vi "Multicast4.vi"(8 "error in":errorcluster, 9 "VersionControl":bool, 11 "type_version":u32 format="%08x") -> (0 "error out":errorcluster, 1 "selDevice":T1, 2 "tblT":string[][](table) caption="Найденные устройства. (Выберите устройство к которому следует подключиться).", 3 "Cancel":bool, 4 "selIPhex":u32 format="%x", 5 "foundDevices":T1[](array[typedef]))   [LabVIEW 2017, in "LV_Unicorn.lvlib"]
uses:
  LV_Unicorn.lvlib
  Control/AnswerUDP.ctl
  <vilib>/Utility/miscctls.llb/LVRowAndColumnTypeDef.ctl
  Common/GlobalMulticast.vi
panel:
  in  "Listbox":i32(listbox)
  in  "Sel":bool
  in  "Cancel":bool
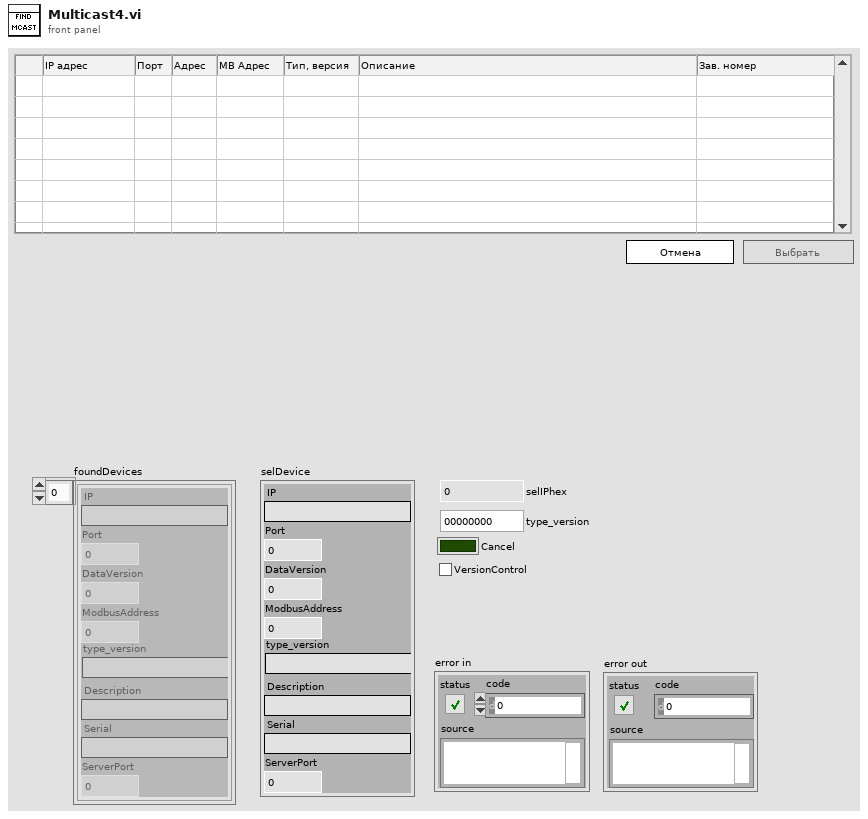
[diagram p1: front panel]
types:
  T1 = typedef "LV_Unicorn.lvlib/AnswerUDP.ctl" = cluster{"IP":string, "Port":u16, "DataVersion":u16, "ModbusAddress":i32, "type_version":string, "Description":string, "Serial":string, "ServerPort":u16}
  T2 = typedef "LVRowAndColumnTypeDef.ctl" = cluster{"Row":i32, "Column":i32}
  T3 = enum8{"Enabled", "Disabled", "Disabled and Grayed Out"}
  T4 = enum32{"Invalid", "Standard", "Closed", "Hidden", "Minimized", "Maximized"}
  T5 = enum32{"Bad", "Idle", "Run top level", "Running"}
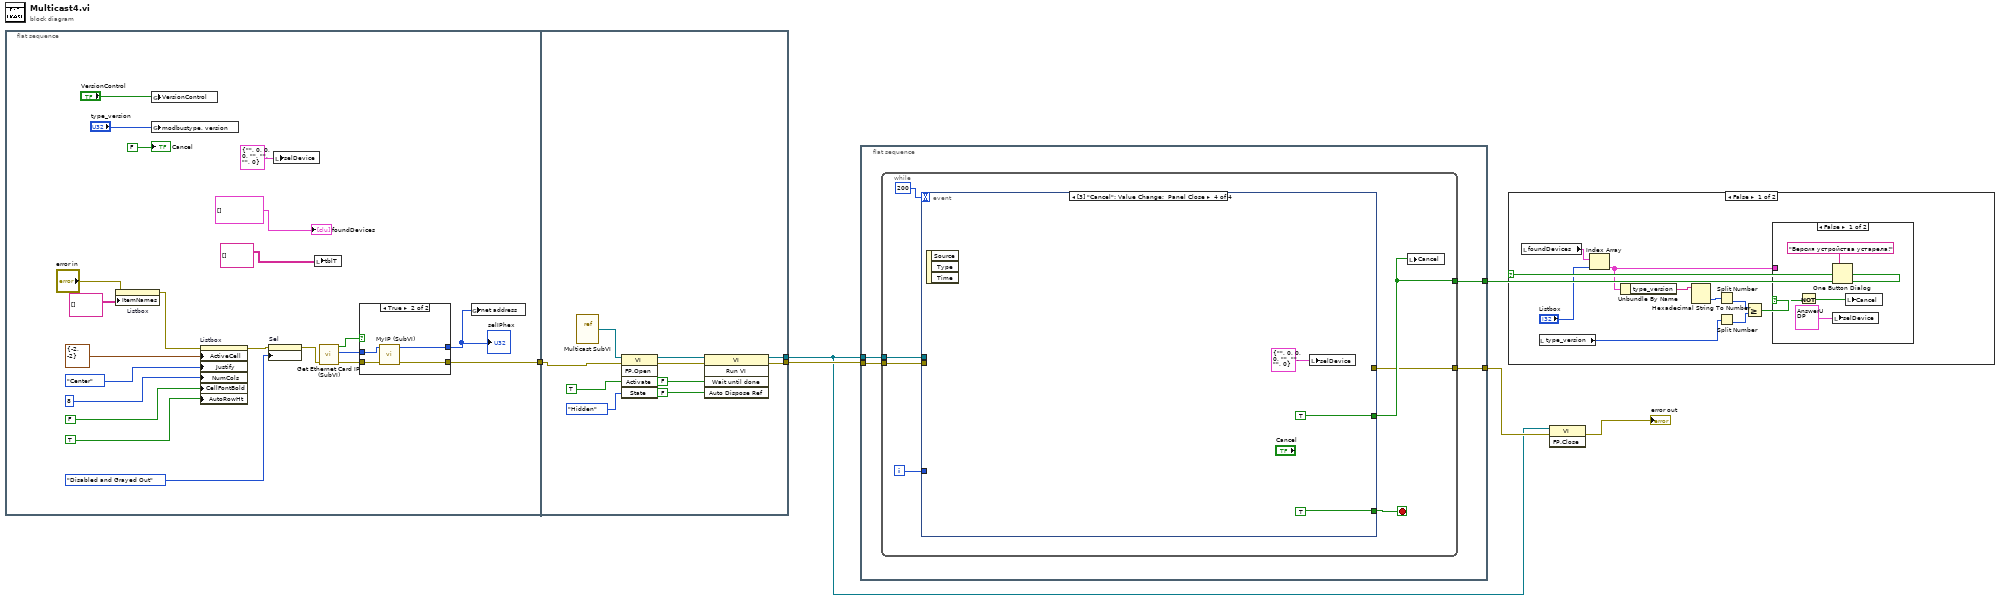
[diagram p0: block diagram]
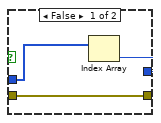
[diagram p2: hidden frame]
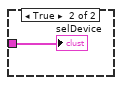
[diagram p3: hidden frame]
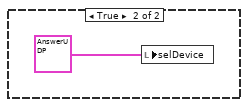
[diagram p4: hidden frame]
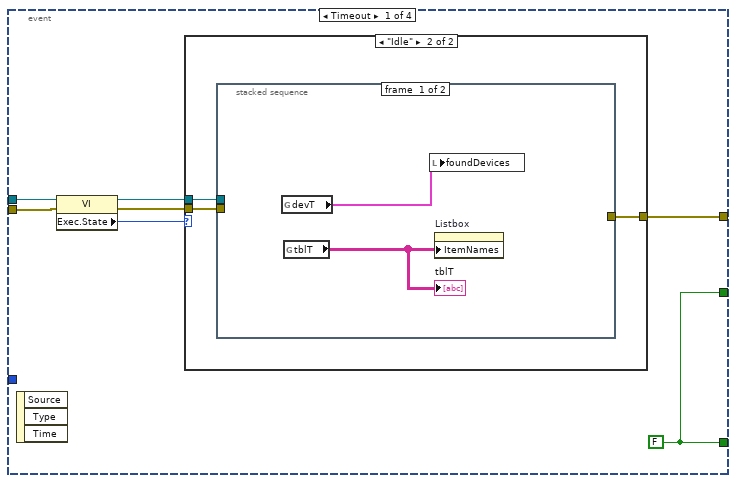
[diagram p5: hidden frame]
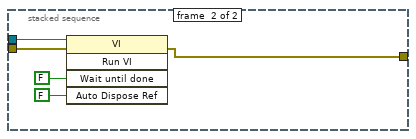
[diagram p7: hidden frame]
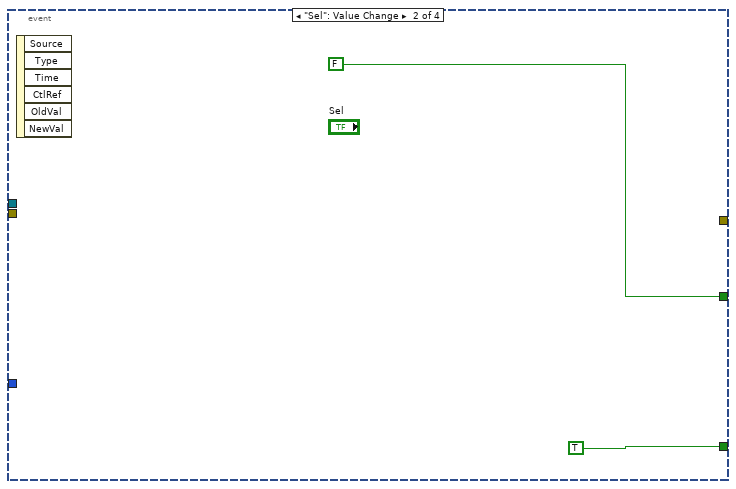
[diagram p8: hidden frame]
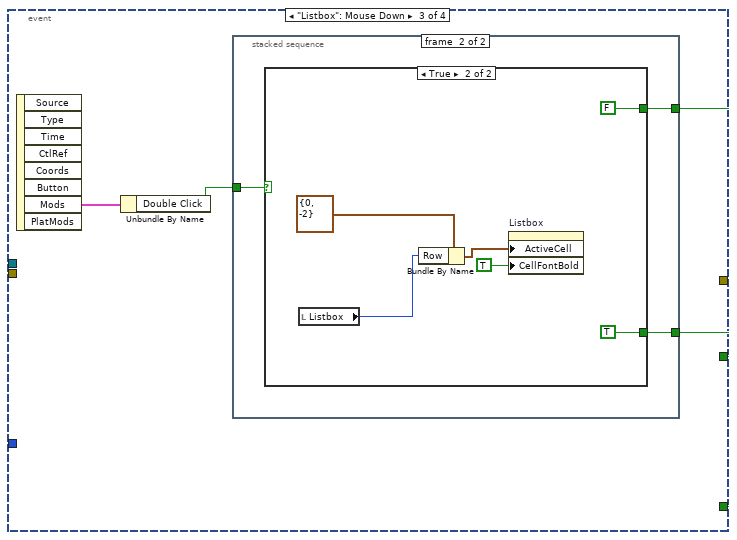
[diagram p9: hidden frame]
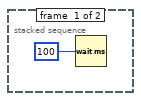
[diagram p10: hidden frame]
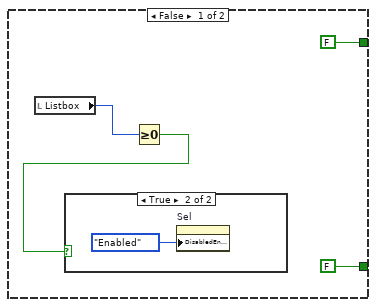
[diagram p11: hidden frame]
diagram:
  n1 = flat-sequence {
    tunnel: [w24] -> w4
    tunnel: [w44] -> w1
    tunnel: [w43] -> w5
    tunnel: w4 -> [w38]
    frame #0 {
      n2 = property on="Listbox" class="MCListbox (strict)"(error in="error in", "ItemNames"=string[][] [] ("Item Names")) -> (error out=w9:errorcluster)  [unwired: 1 in, 1 out]
      n3 = global write "GlobalMulticast.vi" "VersionControl"("VersionControl") -> ()
      n4 = global write "GlobalMulticast.vi" "modbustype, version"("type_version") -> ()
      n5 = property on="Listbox" class="MCListbox (strict)"(error in=w9, "ActiveCell"=T2 {"Row"=-2, "Column"=-2} ("Active Cell:Active Cell"), "Justify"=enum16{"Left", "Center", "Right"}."Center" ("Active Cell:Cell Justification"), "NumCols"=u32 8 ("Number of Columns"), "CellFontBold"=FALSE ("Active Cell:Cell Font:Bold"), "AutoRowHt"=TRUE ("Autosizing Row Height")) -> (error out=w10:errorcluster)  [unwired: 1 in, 1 out]
      n6 = property on="Sel" class="Bool"(error in=w10, "DisabledEnum"=T3."Disabled and Grayed Out" ("Disabled")) -> (error out=w16:errorcluster)  [unwired: 1 in, 1 out]
      n7 = local write "selDevice"(T1 {"IP"="", "Port"=0, "DataVersion"=0, "ModbusAddress"=0, "type_version"="", "Description"="", "Serial"="", "ServerPort"=0} ("selDevicesT")) -> ()
      n8 = local write "tblT"(string[][] [] ("table")) -> ()
      n9 = call "Get Ethernet Card IP (SubVI).vi"("error in (no error)"=w16) -> ("error out"=w28:errorcluster, "IP_hex"=w27:u32[], "FinIPMore1"=w26:bool)  [unwired: 8 in]
      n10 = case shown="True" w26 {
        tunnel: [w30 w33] -> w25
        tunnel: w28 -> [w29 w35]
        tunnel: w27 -> [w31 w34]
        tunnel: [w29 w32] -> w24
        frame False {
          n11 = Index Array(array=w31) -> (element=w30:u32)  [unwired: 1 in]
        }
        frame True {
          n12 = call "MyIP (SubVI).vi"("error in (no error)"=w35, "IPArray"=w34) -> ("error out"=w32:errorcluster, "Sel_IP_hex"=w33:u32)  [unwired: 8 in]
        }
      }
      "selIPhex" <- w25
      n13 = global write "GlobalMulticast.vi" "net address"(w25) -> ()
      "foundDevices" <- T1[] [] ("devices")
      "Cancel" <- FALSE ("Stop")
    }
    frame #1 {
      n14 = vi-ref "Multicast SubVI.vi"() -> (w41:refnum<vi>)
      n15 = invoke class="VI" method="FP.Open"(reference=w41, error in=w38, "Activate"=TRUE ("Activate?"), "State"=T4."Hidden") -> (reference out=w40:refnum<vi>, error out=w39:errorcluster)  [unwired: 1 in, 3 out]
      n16 = invoke class="VI" method="Run VI"(reference=w40, error in=w39, "Wait until done"=FALSE ("Wait Until Done"), "Auto Dispose Ref"=FALSE ("Auto Dispose Reference")) -> (reference out=w44:refnum<vi>, error out=w43:errorcluster)  [unwired: 1 in, 3 out]
    }
  }
  n17 = flat-sequence {
    tunnel: [w49] -> w6
    tunnel: w1 -> [w48]
    tunnel: w5 -> [w47]
    tunnel: [w46] -> w3
    frame #0 {
      n18 = while {
        tunnel: [w54] -> w49
        tunnel: w48 -> [w53]
        tunnel: w47 -> [w52]
        tunnel: [w50] -> w46
        i -> [w55]
        stop <- w56 stop-if-true
        n19 = event shown="[3] \"Cancel\": Value Change;  Panel Close" {
          selector: _ -> [_ _ _ _]
          dyn-events: _ -> [_ _ _ _]
          timeout: 200 -> [_ _ _ _]
          tunnel: [w63 TRUE w79 TRUE] -> w56
          tunnel: w55 -> [_ _ _ _]
          tunnel: [w63 FALSE ("Cancel") w78 TRUE ("Cancel")] -> w54
          tunnel: w53 -> [w62 _ _ _]
          tunnel: w52 -> [w61 _ _ _]
          tunnel: [w57 _ _ _] -> w50
          event Timeout {
            w63 = FALSE
            n20 = event-data() -> ()  [unwired: 1 in, 3 out]
            n21 = property class="VI"(reference=w62, error in=w61) -> (reference out=w58:refnum<vi>, error out=w59:errorcluster, "Exec.State"=w60:T5)
            n22 = case shown="\"Idle\"" w60 {
              tunnel: w59 -> [w64 w67]
              tunnel: w58 -> [_ w66]
              tunnel: [w64 w65] -> w57
              frame "Bad", Default {
              }
              frame "Idle" {
                n23 = stacked-sequence {
                  tunnel: w67 -> [_ w73]
                  tunnel: w66 -> [_ w72]
                  tunnel: [_ w71] -> w65
                  frame #0 {
                    n24 = global read "GlobalMulticast.vi" "devT"() -> (w68:T1[])
                    n25 = global read "GlobalMulticast.vi" "tblT"() -> (w69:string[][])
                    "tblT" <- w69
                    n26 = local write "foundDevices"(w68) -> ()
                    n27 = property on="Listbox" class="MCListbox (strict)"("ItemNames"=w69) -> ()  [unwired: 2 in, 2 out]
                  }
                  frame #1 {
                    n28 = invoke class="VI" method="Run VI"(reference=w72, error in=w73, "Wait until done"=FALSE ("Wait Until Done"), "Auto Dispose Ref"=FALSE ("Auto Dispose Reference")) -> (error out=w71:errorcluster)  [unwired: 1 in, 4 out]
                  }
                }
              }
            }
          }
          event "Sel": Value Change {
            n29 = event-data() -> ()  [unwired: 1 in, 6 out]
          }
          event "Listbox": Mouse Down {
            n30 = event-data() -> ("Mods"=w80:cluster{"Double Click":bool, "Menu Key":bool})  [unwired: 1 in, 7 out]
            n31 = Unbundle By Name(w80) -> ("Double Click"=w77:bool)
            n32 = stacked-sequence {
              tunnel: [_ w84] -> w79
              tunnel: [_ w83] -> w78
              tunnel: w77 -> [_ w82]
              frame #0 {
                n33 = Wait (ms)(milliseconds to wait=u32 100) -> ()  [unwired: 1 out]
              }
              frame #1 {
                n34 = case shown="True" w82 {
                  tunnel: [FALSE TRUE] -> w84
                  tunnel: [FALSE ("Cancel") FALSE ("Cancel")] -> w83
                  frame False {
                    n35 = local read "Listbox"() -> (w86:i32)
                    n36 = Greater Or Equal To 0?(x=w86) -> (x >= 0?=w85:bool)
                    n37 = case shown="True" w85 {
                      frame False {
                      }
                      frame True {
                        n38 = property on="Sel" class="Bool"("DisabledEnum"=T3."Enabled" ("Disabled")) -> ()  [unwired: 2 in, 2 out]
                      }
                    }
                  }
                  frame True {
                    n39 = local read "Listbox"() -> (w92:i32)
                    n40 = Bundle By Name(cluster=T2 {"Row"=0, "Column"=-2} ("Active Cell:Active Cell"), "Row"=w92) -> (w90:T2)
                    n41 = property on="Listbox" class="MCListbox (strict)"("ActiveCell"=w90, "CellFontBold"=TRUE ("Active Cell:Cell Font:Bold")) -> ()  [unwired: 2 in, 2 out]
                  }
                }
              }
            }
          }
          event "Cancel": Value Change; Panel Close {
            n42 = event-data() -> ()  [unwired: 1 in, 3 out]
            n43 = local write "selDevice"(T1 {"IP"="", "Port"=0, "DataVersion"=0, "ModbusAddress"=0, "type_version"="", "Description"="", "Serial"="", "ServerPort"=0} ("selDevicesT")) -> ()
          }
        }
        n44 = local write "Cancel"(w54) -> ()
      }
    }
  }
  n45 = case shown="False" w6 {
    frame False {
      n46 = local read "foundDevices"() -> (w106:T1[])
      n47 = local read "type_version"() -> (w105:u32)
      n48 = Index Array(array=w106, index="Listbox") -> (element=w104:T1)
      n49 = Unbundle By Name(w104) -> ("type_version"=w100:string)
      n50 = Hexadecimal String To Number(string=w100) -> (number=w99:u32)  [unwired: 2 in, 1 out]
      n51 = Split Number(x=w99) -> (lo(x)=w103:u16)  [unwired: 1 out]
      n52 = Split Number(x=w105) -> (lo(x)=w102:u16)  [unwired: 1 out]
      n53 = Greater Or Equal?(x=w103, y=w102) -> (x >= y?=w101:bool)
      n54 = case shown="False" w101 {
        selector: w101 -> [w111 _]
        tunnel: w104 -> [_ w112]
        frame False {
          n55 = Not(x=w111) -> (.not. x?=w110:bool)
          n56 = One Button Dialog(message="Версия устройства устарела!") -> ()  [unwired: 1 in, 1 out]
          n57 = local write "selDevice"(T1 {"IP"="", "Port"=0, "DataVersion"=0, "ModbusAddress"=0, "type_version"="", "Description"="", "Serial"="\u0000\u0000\u0000\u0000\u0000\u0000\u0000\u0000\u0000\u0000\u0000\u0000\u0000\u0000\u0000\u0000\u0000\u0000\u0000\u0000\u0000\u0000\u0000\u0000\u0000\u0000\u0000\u0000\u0000\u0000\u0000\u0000\u0000\u0000\u0000\u0000\u0000", "ServerPort"=0} ("selDevice")) -> ()
          n58 = local write "Cancel"(w110) -> ()
        }
        frame True {
          "selDevice" <- w112
        }
      }
    }
    frame True {
      n59 = local write "selDevice"(T1 {"IP"="", "Port"=0, "DataVersion"=0, "ModbusAddress"=0, "type_version"="", "Description"="", "Serial"="\u0000\u0000\u0000\u0000\u0000\u0000\u0000\u0000\u0000\u0000\u0000\u0000\u0000\u0000\u0000\u0000\u0000\u0000\u0000\u0000\u0000\u0000\u0000\u0000\u0000\u0000\u0000\u0000\u0000\u0000\u0000\u0000\u0000\u0000\u0000\u0000\u0000", "ServerPort"=0} ("selDevice")) -> ()
    }
  }
  n60 = invoke class="VI" method="FP.Close"(reference=w1, error in=w3) -> (error out=→"error out":errorcluster)  [unwired: 1 in, 2 out]
